vi "niRFUtil RFHS Math Apply Polynomial CSG.vi"(0 "X":sgl[](array[numeric]), 5 "P(A)":csg[](array[numeric]), 11 "error in":errorcluster) -> (4 "P(x)":csg[](array[numeric]), 15 "error out":errorcluster)   [LabVIEW 2015, in "niRFUtil.lvlib"]
uses:
  niRFUtil.lvlib
panel:
  out "elapsedTime":sgl
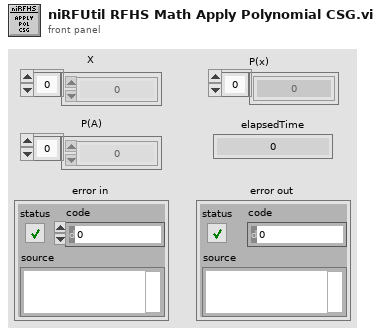
[diagram p1: front panel]
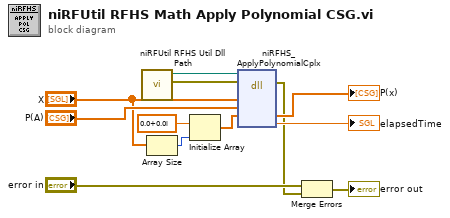
[diagram p0: block diagram]
diagram:
  n1 = call "niRFUtil RFHS Util Dll Path.vi"() -> ("error out"=w2:errorcluster, "Path"=w6:path)  [unwired: 7 in, 3 out]
  n2 = Array Size(array="X") -> (size(s)=w3:i32)
  n3 = Initialize Array(csg 0.0+0.0i ("dimension size"), w3) -> (w5:csg[])
  n4 = dll-call lib="R:/niRFHS.dll" fn="niRFHS_ApplyPolynomialCplx"(path in=w6, error in=w2, "input"="X", "polynom"="P(A)", "output"=w5) -> (error out=w1:errorcluster, "output"=→"P(x)":csg[], "elapsedTime"=→"elapsedTime":sgl)  [unwired: 5 in, 1 out]
  n5 = Merge Errors("error in", w1) -> (→"error out":errorcluster)
